vi "cg_fid_V1.1.vi"() -> ()   [LabVIEW 2011]
panel:
  out "Integral":dbl
  out "Time (min)":dbl
  out "Numeric":i32
  in  "Stop Time (min)":dbl=15.0
  out "Time has Elapsed":bool
  in  "Start Button":bool
  out "TCD":dbl(graph)
  out "FID":dbl(graph)
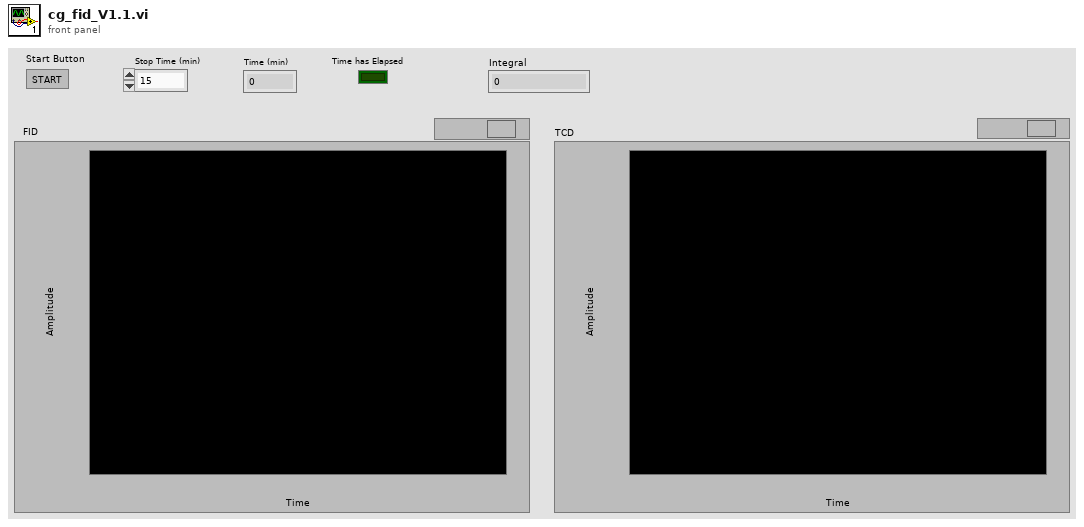
[diagram p1: front panel]
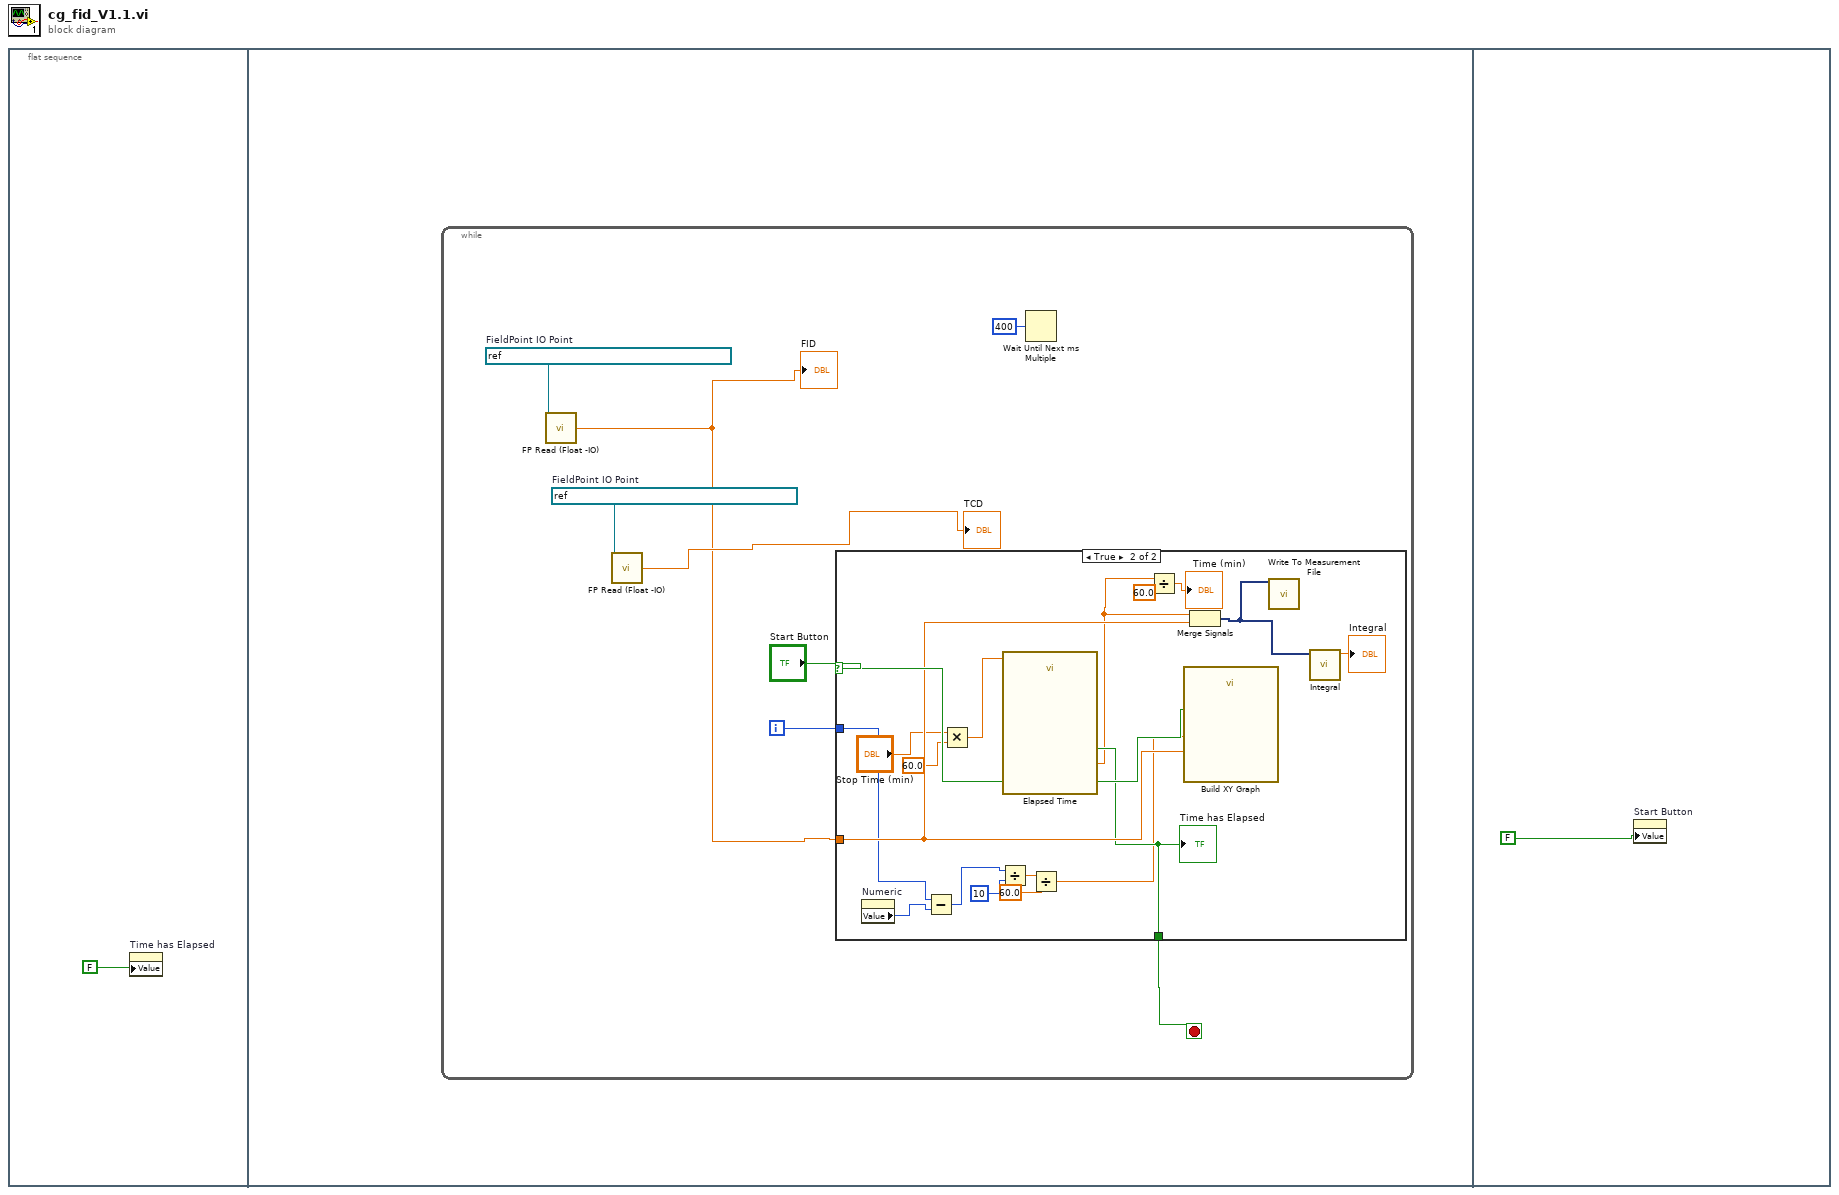
[diagram p0: block diagram]
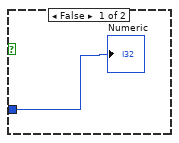
[diagram p2: hidden frame]
diagram:
  n1 = flat-sequence {
    frame #0 {
      n2 = property on="Time has Elapsed" class="Bool (strict)"("Value"=FALSE) -> ()  [unwired: 2 in, 2 out]
    }
    frame #1 {
      n3 = while {
        i -> [w2]
        stop <- w3 stop-if-true
        w8 = refnum<k21> "FieldPoint\\cfp2220\\cFP-AI-110 @4\\Channel 2"  # FieldPoint IO Point
        w9 = refnum<k21> "FieldPoint\\cfp2220\\cFP-AI-110 @4\\Channel 0"  # FieldPoint IO Point
        n4 = call <vilib>:"FP Read (Float -IO).vi"("FieldPoint IO Point In"=w9) -> ("value"=w4:dbl)  [unwired: 11 in, 3 out]
        "FID" <- w4
        n5 = call <vilib>:"FP Read (Float -IO).vi"("FieldPoint IO Point In"=w8) -> ("value"=→"TCD":dbl)  [unwired: 11 in, 3 out]
        n6 = case shown="True" "Start Button" {
          selector: "Start Button" -> [_ w28]
          tunnel: w4 -> [_ w27]
          tunnel: [_ w26] -> w3
          tunnel: w2 -> [w10 w21]
          frame False {
            "Numeric" <- w10
          }
          frame True {
            n7 = property on="Numeric" class="DigNum (strict)"() -> ("Value"=w20:i32)  [unwired: 2 in, 2 out]
            n8 = Subtract(x=w21, y=w20) -> (x-y=w22:i32)
            n9 = Multiply(x="Stop Time (min)", y=60.0) -> (x*y=w18:dbl)
            n10 = Divide(x=w22, y=10) -> (x/y=w24:dbl)
            n11 = call "Elapsed Time"("Time Target (s)"=w18) -> ("Elapsed Time (s)"=w13:dbl, "Time has Elapsed"=w26:bool)  [unwired: 11 in, 6 out]
            "Time has Elapsed" <- w26
            n12 = Divide(x=w24, y=60.0) -> (x/y=w19:dbl)
            n13 = Divide(x=w13, y=60.0) -> (x/y=→"Time (min)":dbl)
            n14 = call "Build XY Graph"("Enable"=w28, "Y Input"=w27, "X Input"=w19) -> ()  [unwired: 2 in, 7 out]
            n15 = Merge Signals(w13, w27) -> (w12:dynamicdata)
            n16 = call "Write To Measurement File"("Signals"=w12) -> ()  [unwired: 16 in, 3 out]
            n17 = call "Integral.vi"("Tested Signals"=w12) -> ("Integral"=→"Integral":dbl)  [unwired: 9 in, 1 out]
          }
        }
        n18 = Wait Until Next ms Multiple(millisecond multiple=u32 400) -> ()  [unwired: 1 out]
      }
    }
    frame #2 {
      n19 = property on="Start Button" class="Bool (strict)"("Value"=FALSE) -> ()  [unwired: 2 in, 2 out]
    }
  }
